vi "windup&&controlSignal.vi"(9 "error":dbl, 10 "u2k":dbl, 11 "uk":dbl) -> (2 "uk":dbl, 3 "u2k":dbl)   [LabVIEW 2019]
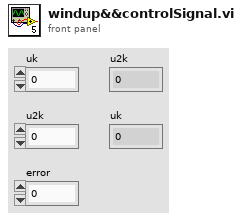
[diagram p1: front panel]
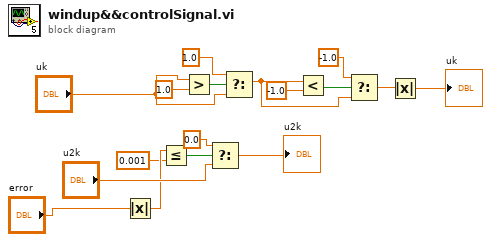
[diagram p0: block diagram]
diagram:
  n1 = Absolute Value(x="error") -> (abs(x)=w15:dbl)
  n2 = Less Or Equal?(x=w15, y=0.001) -> (x <= y?=w12:bool)
  n3 = Greater?(x="uk", y=1.0) -> (0:w2:bool)
  n4 = Select(t=0.0, s=w12, f="u2k") -> (s? t:f=→"u2k":dbl)
  n5 = Select(t=1.0, s=w2, f="uk") -> (s? t:f=w9:dbl)
  n6 = Less?(x=w9, y=-1.0) -> (x < y?=w7:bool)
  n7 = Select(t=-1.0, s=w7, f=w9) -> (s? t:f=w10:dbl)
  n8 = Absolute Value(x=w10) -> (abs(x)=→"uk":dbl)
